vi "Color Map Store.vi"(7 "Mode":T1, 8 "Error In":errorcluster, 11 "colorMap":string) -> (0 "Error Out":errorcluster, 2 "colorMap String":string, 3 "colorMap":T2[](array[typedef]))   [LabVIEW 2019, in "LSS.lvlib"]
doc: "This functional global variable stores the color map values so other LSS functions can make sure of those values without needing to pass in the color map values with each LSS string.\n\n<b>Inputs:</b>\n<b>colorMap</b> - This string is an LSS formatted string that allows the mapping of hexidecimal color constants to string names that are easier to remember. Once a color is defined in the colorMap, any subsequent LSS call can simply use the name of the color instead of the hexidecimal representation. This input is only used when the mode input is set to \"Write\" or \"Add\". The format for this string is as follows:\n colorMap{\n myColorName:#000000;\n }\n<b>Mode</b> - Select between the following options:\n1. Write - Saves the colorMap input string for use by later LSS functions. Will overwrite any previously saved colormap values.\n2. Add - Adds the new colorMap LSS string to the existing string.\n3. Read - Reads all currently saved color map values.\n<b>Error In</b> - Error input terminal\n\n<b>Outputs:</b>\n<b>colorMap</b> - Contains the data from the colorMap input string as a parsed array that is used by LSS functions for changing style of the UI.\n<b>colorMap String</b> - Outputs the text of the items saved in the color map as a string.\n<b>Error Out</b> - Error output terminal"
uses:
  LSS.lvlib
  Controls/colorMap.ctl
  Controls/Mode.ctl
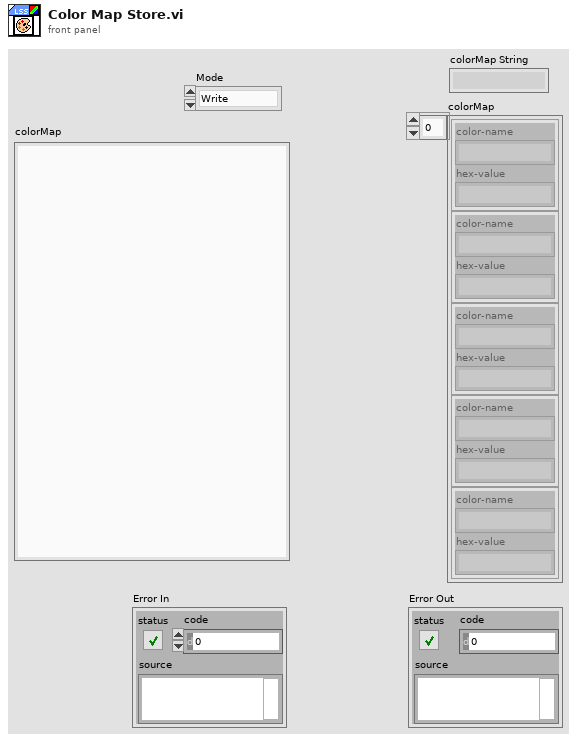
[diagram p1: front panel]
types:
  T1 = typedef "LSS.lvlib/Mode.ctl" = enum16{"Write", "Add", "Read"}
  T2 = typedef "LSS.lvlib/colorMap.ctl" = cluster{"color-name":string, "hex-value":string}
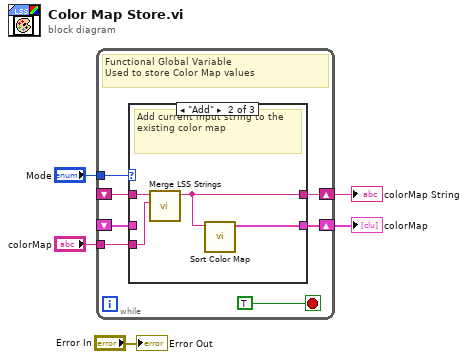
[diagram p0: block diagram]
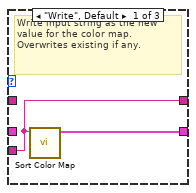
[diagram p2: hidden frame]
diagram:
  n1 = while {
    tunnel: "colorMap" -> [w10]
    tunnel: "Mode" -> [w11]
    shift-right: [w9] -> w3
    shift-left: _ -> [w8]
    shift-right: [w7] -> w1
    shift-left: _ -> [w6]
    stop <- TRUE stop-if-true
    # "Functional Global Variable\nUsed to store Color Map values"
    n2 = case shown="\"Add\"" w11 {
      tunnel: w10 -> [w13 w17 _]
      tunnel: [w14 w16 w20] -> w9
      tunnel: w8 -> [_ _ w20]
      tunnel: [w13 w15 w19] -> w7
      tunnel: w6 -> [_ w18 w19]
      frame "Write", Default {
        # "Write input string as the new value for the color map. Overwrites existing if any."
        n3 = call "Sort Color Map.vi"("colorMap"=w13) -> ("Parsed Color Map"=w14:T2[])  [unwired: 10 in]
      }
      frame "Add" {
        # "Add current input string to the existing color map"
        n4 = call "Merge LSS Strings.vi"("Merge String"=w17, "LSS Before"=w18) -> ("LSS After"=w15:string)  [unwired: 9 in]
        n5 = call "Sort Color Map.vi"("colorMap"=w15) -> ("Parsed Color Map"=w16:T2[])  [unwired: 10 in]
      }
      frame "Read" {
        # "Read stored color map values"
      }
    }
  }
  "colorMap" <- w3
  "colorMap String" <- w1
  "Error Out" <- "Error In"
